vi "CalculateFeedForwardIIRcoeffs.vi"(10 "fs [MHz]":dbl, 11 "fc [MHz]":dbl) -> (0 "a1":dbl, 1 "b2":dbl, 2 "b1":dbl, 3 "b0":dbl, 4 "a2":dbl)   [LabVIEW 2018]
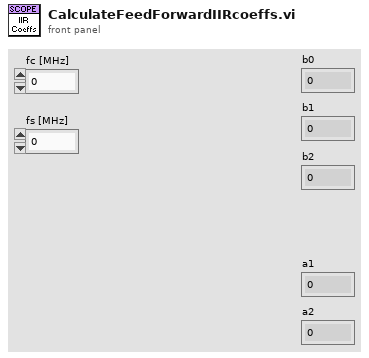
[diagram p1: front panel]
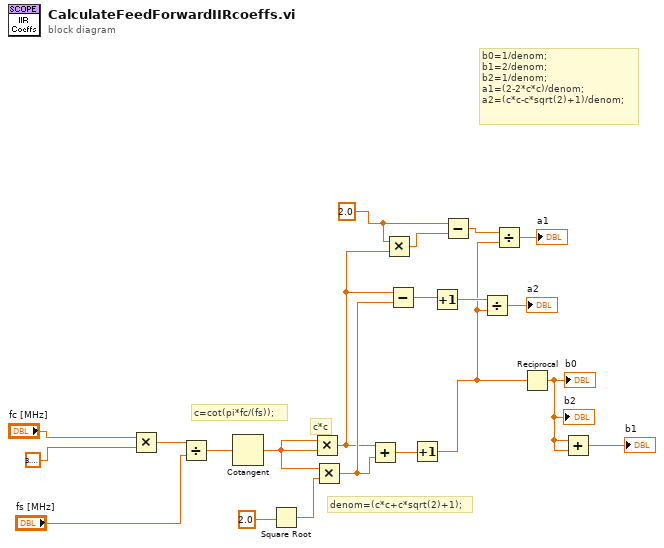
[diagram p0: block diagram]
diagram:
  w5 = 2.0
  # "c*c"
  # "b0=1/denom;\nb1=2/denom;\nb2=1/denom;\na1=(2-2*c*c)/denom; \na2=(c*c-c*sqrt(2)+1)/denom;"
  # "c=cot(pi*fc/(fs));"
  # "denom=(c*c+c*sqrt(2)+1);"
  n1 = Multiply(x="fc [MHz]", y=3.141592653589793) -> (x*y=w19:dbl)
  n2 = Divide(x=w19, y="fs [MHz]") -> (x/y=w17:dbl)
  n3 = Cotangent(1:w17) -> (0:w15:dbl)
  n4 = Square Root(x=2.0) -> (sqrt(x)=w14:dbl)
  n5 = Multiply(x=w15, y=w15) -> (x*y=w6:dbl)
  n6 = Multiply(x=w15, y=w14) -> (x*y=w10:dbl)
  n7 = Add(x=w6, y=w10) -> (x+y=w13:dbl)
  n8 = Multiply(x=w5, y=w6) -> (x*y=w4:dbl)
  n9 = Subtract(x=w6, y=w10) -> (x-y=w9:dbl)
  n10 = Increment(x=w13) -> (x+1=w2:dbl)
  n11 = Increment(x=w9) -> (x+1=w8:dbl)
  n12 = Subtract(x=w5, y=w4) -> (x-y=w3:dbl)
  n13 = Divide(x=w8, y=w2) -> (x/y=→"a2":dbl)
  n14 = Divide(x=w3, y=w2) -> (x/y=→"a1":dbl)
  n15 = Reciprocal(x=w2) -> (1/x=w12:dbl)
  "b0" <- w12
  "b2" <- w12
  n16 = Add(x=w12, y=w12) -> (x+y=→"b1":dbl)
